vi "I8_1D.vi"(4 "Value":T1) -> (1 "Constant":refnum<class "Const_I16_1D.lvclass">)   [LabVIEW 2021, in "Const_I16_1D.lvclass"]
uses:
  Const_I16_1D.lvclass
  Type.ctl
  Const_I16_1D.lvclass/Const_I16_1D.ctl
  Properties/Write Value.vi
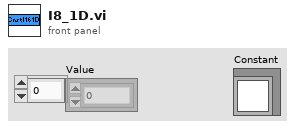
[diagram p1: front panel]
types:
  T1 = typedef "Const_I16_1D.lvclass/Type.ctl" = i16[]
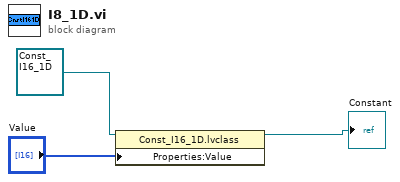
[diagram p0: block diagram]
diagram:
  n1 = property class="Const_I16_1D.lvclass"(reference=refnum<class "Const_I16_1D.lvclass"> refnum ("Constants.lvlib:Numeric.lvclass"), "Properties:Value"="Value") -> (reference out=→"Constant":refnum<class "Const_I16_1D.lvclass">)  [unwired: 1 in, 1 out]
